vi "log analysis_gps.vi"() -> ()   [LabVIEW 2019] (continued)
2107,281532.450,02000000,471d,15824;INS_ALIGNMENT_COMPLETE,INS_RTKFIXED,37.37125529086,126.72205393210,7.8208,22.3000,-0.0380,0.2964,0.0024,-1.066354382,0.654899534,89.120116128,0.4138,0.2906,0.5321,0.1104,0.0921,0.0766,0.1807,0.1849,5.1689,0f000001,0*be946886\n\t", "INSPVAXA,USB3,0,47.5,FINESTEERING,2107,281532.950,02000000,471d,15824;INS_ALIGNMENT_COMPLETE,INS_RTKFIXED,37.37125523061,126.72205555403,7.8287,22.3000,-0.0378,0.2817,0.0049,-1.169453281,0.642583735,89.146408526,0.4138,0.2906,0.5321,0.1104,0.0921,0.0766,0.1807,0.1849,5.1689,0f000001,0*6f8607ae\n\t", "INSPVAXA,USB3,0,48.5,FINESTEERING,2107,281533.450,02000000,471d,15824;INS_ALIGNMENT_COMPLETE,INS_RTKFIXED,37.37125517665,126.72205724840,7.8341,22.3000,-0.0370,0.2921,0.0139,-1.096637131,0.532202635,89.160335545,0.4113,0.2846,0.5267,0.1101,0.0906,0.0761,0.1804,0.1849,5.1704,0f000001,0*30c8b167\n\t", "INSPVAXA,USB3,0,48.5,FINESTEERING,2107,281533.950,02000000,471d,15824;INS_ALIGNMENT_COMPLETE,INS_RTKFIXED,37.37125511841,126.72205890911,7.8393,22.3000,-0.0280,0.2944,0.0195,-1.130148525,0.576717755,89.139209909,0.4113,0.2846,0.5267,0.1101,0.0906,0.0761,0.1804,0.1849,5.1704,0f000001,0*9cf16a0c\n\t", "INSPVAXA,USB3,0,49.0,FINESTEERING,2107,281534.450,02000000,471d,15824;INS_ALIGNMENT_COMPLETE,INS_RTKFIXED,37.37125507853,126.72206052520,7.8451,22.3000,-0.0278,0.2839,0.0233,-1.120245446,0.696634414,89.152346595,0.4098,0.2808,0.5226,0.1101,0.0900,0.0757,0.1802,0.1849,5.1715,0f000001,0*4ae7b9de\n\t", "INSPVAXA,USB3,0,48.5,FINESTEERING,2107,281535.450,02000000,471d,15824;INS_ALIGNMENT_COMPLETE,INS_RTKFIXED,37.37125500223,126.72206378998,7.8595,22.3000,-0.0263,0.2848,0.0309,-1.021616386,0.668311678,89.031237589,0.4086,0.2786,0.5193,0.1098,0.0898,0.0755,0.1801,0.1849,5.1718,0f000001,0*96cd35cb\n\t", "INSPVAXA,USB3,0,48.5,FINESTEERING,2107,281535.950,02000000,471d,15824;INS_ALIGNMENT_COMPLETE,INS_RTKFIXED,37.37125496736,126.72206538562,7.8673,22.3000,-0.0208,0.2826,0.0283,-0.984984816,0.649258027,88.926389870,0.4086,0.2786,0.5193,0.1098,0.0898,0.0755,0.1801,0.1849,5.1718,0f000001,0*d651761b\n\t", "INSPVAXA,USB3,0,43.0,FINESTEERING,2107,281536.450,02000000,471d,15824;INS_ALIGNMENT_COMPLETE,INS_RTKFIXED,37.37125494902,126.72206698066,7.8731,22.3000,-0.0263,0.2809,0.0211,-1.040366850,0.673880913,88.812825832,0.4080,0.2774,0.5168,0.1098,0.0898,0.0754,0.1801,0.1849,5.1719,0f000001,0*bc17f841\n\t", "INSPVAXA,USB3,0,43.0,FINESTEERING,2107,281536.950,02000000,471d,15824;INS_ALIGNMENT_COMPLETE,INS_RTKFIXED,37.37125492336,126.72206864315,7.8782,22.3000,-0.0243,0.2721,0.0164,-1.054954219,0.518295221,88.745495992,0.4080,0.2774,0.5168,0.1098,0.0898,0.0754,0.1801,0.1849,5.1719,0f000001,0*93a4c9d5\n\t", "INSPVAXA,USB3,0,49.5,FINESTEERING,2107,281537.450,02000000,471d,15824;INS_ALIGNMENT_COMPLETE,INS_RTKFIXED,37.37125492115,126.72207026375,7.8826,22.3000,-0.0312,0.2819,0.0093,-1.140326521,0.505680826,88.594443704,0.4075,0.2769,0.5150,0.1098,0.0900,0.0754,0.1800,0.1848,5.1716,0f000001,0*0036ae1b\n\t", "INSPVAXA,USB3,0,49.5,FINESTEERING,2107,281537.950,02000000,471d,15824;INS_ALIGNMENT_COMPLETE,INS_RTKFIXED,37.37125491697,126.72207184054,7.8872,22.3000,-0.0272,0.2819,0.0040,-1.130976236,0.507935776,88.476377303,0.4075,0.2769,0.5150,0.1098,0.0900,0.0754,0.1800,0.1848,5.1716,0f000001,0*f6fa546b\n\t", "INSPVAXA,USB3,0,49.5,FINESTEERING,2107,281538.450,02000000,471d,15824;INS_ALIGNMENT_COMPLETE,INS_RTKFIXED,37.37125491162,126.72207343326,7.8918,22.3000,-0.0245,0.2815,0.0124,-1.153453506,0.493104111,88.435314047,0.4072,0.2765,0.5135,0.1099,0.0900,0.0754,0.1800,0.1848,5.1710,0f000001,0*5ae8f9c6\n\t", "INSPVAXA,USB3,0,49.5,FINESTEERING,2107,281538.950,02000000,471d,15824;INS_ALIGNMENT_COMPLETE,INS_RTKFIXED,37.37125490028,126.72207504818,7.8968,22.3000,-0.0236,0.2833,0.0059,-1.091251980,0.482969465,88.379863366,0.4072,0.2765,0.5135,0.1099,0.0900,0.0754,0.1800,0.1848,5.1710,0f000001,0*2ba689f0\n\t", "INSPVAXA,USB3,0,48.5,FINESTEERING,2107,281539.450,02000000,471d,15824;INS_ALIGNMENT_COMPLETE,INS_RTKFIXED,37.37125490824,126.72207664117,7.9004,22.3000,-0.0216,0.2784,0.0079,-1.109314476,0.482411091,88.340192961,0.4069,0.2763,0.5124,0.1098,0.0900,0.0754,0.1799,0.1848,5.1698,0f000001,0*8761aced\n\t", "INSPVAXA,USB3,0,48.5,FINESTEERING,2107,281539.950,02000000,471d,15824;INS_ALIGNMENT_COMPLETE,INS_RTKFIXED,37.37125492237,126.72207822482,7.9044,22.3000,-0.0192,0.2821,0.0128,-1.302544684,0.456729396,88.350488881,0.4069,0.2763,0.5124,0.1098,0.0900,0.0754,0.1799,0.1848,5.1698,0f000001,0*d36670cb\n\t", "INSPVAXA,USB3,0,49.0,FINESTEERING,2107,281540.450,02000000,471d,15824;INS_ALIGNMENT_COMPLETE,INS_RTKFIXED,37.37125492050,126.72207986895,7.9075,22.3000,-0.0253,0.2731,0.0097,-1.293452361,0.411042124,88.411048342,0.4069,0.2763,0.5116,0.1099,0.0902,0.0754,0.1799,0.1848,5.1684,0f000001,0*2b0ddc64\n\t", "INSPVAXA,USB3,0,48.5,FINESTEERING,2107,281541.950,02000000,471d,15824;INS_ALIGNMENT_COMPLETE,INS_RTKFIXED,37.37125486975,126.72208463852,7.9183,22.3000,-0.0254,0.2525,0.0080,-1.001794555,0.208047593,88.595435121,0.4068,0.2761,0.5109,0.1098,0.0900,0.0754,0.1799,0.1848,5.1663,0f000001,0*dcb79567\n\t", "INSPVAXA,USB3,0,49.0,FINESTEERING,2107,281542.450,02000000,471d,15824;INS_ALIGNMENT_COMPLETE,INS_RTKFIXED,37.37125484773,126.72208610696,7.9206,22.3000,-0.0083,0.3427,0.0268,-0.912942470,0.207155867,88.931332893,0.4067,0.2761,0.5105,0.1096,0.0899,0.0754,0.1798,0.1848,5.1642,0f000001,0*e5dcf027\n\t", "INSPVAXA,USB3,0,49.5,FINESTEERING,2107,281543.950,02000000,471d,15824;INS_ALIGNMENT_COMPLETE,INS_RTKFIXED,37.37125492276,126.72209111825,7.9296,22.3000,0.0316,0.2804,0.0153,-0.692370784,0.020659336,82.875038153,0.4068,0.2761,0.5102,0.1095,0.0899,0.0754,0.1798,0.1847,5.1628,0f000001,0*67f5d293\n\t", "INSPVAXA,USB3,0,50.0,FINESTEERING,2107,281544.450,02000000,471d,15824;INS_ALIGNMENT_COMPLETE,INS_RTKFIXED,37.37125505566,126.72209271509,7.9316,22.3000,0.0505,0.2738,0.0268,-0.616767786,0.154143258,78.067707223,0.4067,0.2763,0.5098,0.1099,0.0900,0.0754,0.1797,0.1847,5.1619,0f000001,0*4337cbac\n\t", "INSPVAXA,USB3,0,47.5,FINESTEERING,2107,281545.450,02000000,471d,15824;INS_ALIGNMENT_COMPLETE,INS_RTKFIXED,37.37125567911,126.72209586319,7.9361,22.3000,0.0734,0.2704,0.0174,-0.731540413,0.133149102,70.486374677,0.4064,0.2767,0.5097,0.1103,0.0911,0.0753,0.1798,0.1847,5.1599,0f000001,0*4759ac49\n\t", "INSPVAXA,USB3,0,47.5,FINESTEERING,2107,281545.950,02000000,471d,15824;INS_ALIGNMENT_COMPLETE,INS_RTKFIXED,37.37125607129,126.72209738757,7.9408,22.3000,0.0944,0.2605,0.0183,-0.696019275,0.088406772,68.352521751,0.4064,0.2767,0.5097,0.1103,0.0911,0.0753,0.1798,0.1847,5.1599,0f000001,0*d303d9f5\n\t", "INSPVAXA,USB3,0,49.0,FINESTEERING,2107,281546.450,02000000,471d,15824;INS_ALIGNMENT_COMPLETE,INS_RTKFIXED,37.37125652974,126.72209892700,7.9445,22.3000,0.1147,0.2632,0.0224,-0.803440869,0.020202834,66.760557028,0.4064,0.2770,0.5100,0.1115,0.0928,0.0753,0.1798,0.1846,5.1557,0f000001,0*6d000163\n\t", "INSPVAXA,USB3,0,51.5,FINESTEERING,2107,281547.950,02000000,471d,15824;INS_ALIGNMENT_COMPLETE,INS_RTKFIXED,37.37125797695,126.72210352475,7.9421,22.3000,0.1103,0.2645,0.0073,-1.143829533,0.094704547,65.656045982,0.4068,0.2775,0.5101,0.1136,0.0952,0.0753,0.1797,0.1843,5.1506,0f000001,0*3e76ed6a\n\t", "INSPVAXA,USB3,0,46.5,FINESTEERING,2107,281548.450,02000000,471d,15824;INS_ALIGNMENT_COMPLETE,INS_RTKFIXED,37.37125842194,126.72210499734,7.9414,22.3000,0.0987,0.2565,0.0113,-1.211419516,0.114110023,65.814844612,0.4000,0.2752,0.5002,0.1145,0.0964,0.0745,0.1794,0.1832,5.1447,0f000001,0*e7619ae9\n\t", "INSPVAXA,USB3,0,50.0,FINESTEERING,2107,281550.450,02000000,471d,15824;INS_ALIGNMENT_COMPLETE,INS_RTKFIXED,37.37126014909,126.72211137085,7.9382,22.3000,0.0775,0.2990,0.0098,-1.324688179,-0.327901204,70.475818892,0.4093,0.2808,0.5055,0.1189,0.0988,0.0751,0.1779,0.1804,5.1364,0f000001,0*808235da\n\t", "INSPVAXA,USB3,0,50.0,FINESTEERING,2107,281550.950,02000000,471d,15824;INS_ALIGNMENT_COMPLETE,INS_RTKFIXED,37.37126045851,126.72211301062,7.9366,22.3000,0.0692,0.2949,0.0149,-1.528450256,-0.256130387,73.623851068,0.4093,0.2808,0.5055,0.1189,0.0988,0.0751,0.1779,0.1804,5.1364,0f000001,0*9b441f42\n\t", "INSPVAXA,USB3,0,50.5,FINESTEERING,2107,281551.450,02000000,471d,15824;INS_ALIGNMENT_COMPLETE,INS_RTKFIXED,37.37126071585,126.72211464730,7.9349,22.3000,0.0461,0.2986,0.0130,-1.521992533,-0.266379838,76.609836903,0.4123,0.2823,0.5064,0.1185,0.0974,0.0752,0.1766,0.1780,5.1359,0f000001,0*10c7b170\n\t", "INSPVAXA,USB3,0,46.0,FINESTEERING,2107,281553.450,02000000,471d,15824;INS_ALIGNMENT_COMPLETE,INS_RTKFIXED,37.37126103128,126.72212124839,7.9298,22.3000,-0.0140,0.3127,0.0103,-1.123324065,0.508186608,86.475443339,0.4150,0.2827,0.5081,0.1139,0.0931,0.0752,0.1739,0.1735,5.1368,0f000001,0*51a33212\n\t", "INSPVAXA,USB3,0,46.0,FINESTEERING,2107,281553.950,02000000,471d,15824;INS_ALIGNMENT_COMPLETE,INS_RTKFIXED,37.37126097435,126.72212290595,7.9280,22.3000,-0.0108,0.3087,0.0193,-0.994058231,0.235221833,88.104277640,0.4150,0.2827,0.5081,0.1139,0.0931,0.0752,0.1739,0.1735,5.1368,0f000001,0*a2074ee6\n\t", "INSPVAXA,USB3,0,47.5,FINESTEERING,2107,281557.450,02000000,471d,15824;INS_ALIGNMENT_COMPLETE,INS_RTKFIXED,37.37126007127,126.72213399175,7.9228,22.3000,-0.0436,0.2932,0.0085,-0.364989974,-0.412142636,90.870623018,0.4100,0.2787,0.5090,0.1093,0.0914,0.0751,0.1708,0.1703,5.1179,0f000001,0*5c4f0bd9\n\t", "INSPVAXA,USB3,0,46.0,FINESTEERING,2107,281558.450,02000000,471d,15824;INS_ALIGNMENT_COMPLETE,INS_RTKFIXED,37.37125980811,126.72213741354,7.9201,22.3000,-0.0396,0.2827,0.0144,-0.665732137,-0.749833579,90.834139291,0.4087,0.2784,0.5089,0.1102,0.0917,0.0750,0.1706,0.1703,5.1108,0f000001,0*c48606ec\n\t", "INSPVAXA,USB3,0,46.0,FINESTEERING,2107,281558.950,02000000,471d,15824;INS_ALIGNMENT_COMPLETE,INS_RTKFIXED,37.37125968631,126.72213896635,7.9182,22.3000,-0.0389,0.2938,0.0155,-0.920394419,-0.718289974,90.450245046,0.4087,0.2784,0.5089,0.1102,0.0917,0.0750,0.1706,0.1703,5.1108,0f000001,0*246e9289\n\t", "INSPVAXA,USB3,0,48.5,FINESTEERING,2107,281582.000,02000000,471d,15824;INS_ALIGNMENT_COMPLETE,INS_RTKFIXED,37.37125926697,126.72221314243,7.9638,22.3000,0.0065,0.2832,0.0220,-0.844956483,-0.026158862,84.896486231,0.4081,0.2757,0.5033,0.1092,0.0895,0.0749,0.1683,0.1693,5.0877,0f000001,0*999c2cb4\n\t", "INSPVAXA,USB3,0,45.5,FINESTEERING,2107,281585.000,02000000,471d,15824;INS_ALIGNMENT_COMPLETE,INS_RTKFIXED,37.37125940272,126.72222284495,7.9649,22.3000,-0.0095,0.2865,0.0182,-0.747268326,0.234159981,85.317572401,0.4076,0.2752,0.5032,0.1094,0.0898,0.0748,0.1683,0.1693,5.0921,0f000001,0*05cc0da4\n\t", "INSPVAXA,USB3,0,49.5,FINESTEERING,2107,281585.500,02000000,471d,15824;INS_ALIGNMENT_COMPLETE,INS_RTKFIXED,37.37125941547,126.72222448778,7.9662,22.3000,-0.0142,0.2884,0.0124,-0.699076432,0.369703687,85.497806859,0.4078,0.2753,0.5032,0.1096,0.0899,0.0748,0.1684,0.1693,5.0937,0f000001,0*7e52f1b7\n\t", "INSPVAXA,USB3,0,49.5,FINESTEERING,2107,281586.500,02000000,471d,15824;INS_ALIGNMENT_COMPLETE,INS_RTKFIXED,37.37125940571,126.72222789541,7.9680,22.3000,0.0030,0.3079,0.0233,-0.562980027,0.263238278,85.915106652,0.4081,0.2752,0.5032,0.1097,0.0899,0.0748,0.1684,0.1692,5.0953,0f000001,0*7d04a5bf\n\t", "INSPVAXA,USB3,0,49.5,FINESTEERING,2107,281587.000,02000000,471d,15824;INS_ALIGNMENT_COMPLETE,INS_RTKFIXED,37.37125938358,126.72222955995,7.9677,22.3000,-0.0088,0.3126,0.0171,-0.528697229,0.195556365,86.199096589,0.4081,0.2752,0.5032,0.1097,0.0899,0.0748,0.1684,0.1692,5.0953,0f000001,0*98856aba\n\t", "INSPVAXA,USB3,0,47.0,FINESTEERING,2107,281587.500,02000000,471d,15824;INS_ALIGNMENT_COMPLETE,INS_RTKFIXED,37.37125935739,126.72223128487,7.9668,22.3000,-0.0030,0.3090,0.0190,-0.470354496,0.052583887,86.493869068,0.4079,0.2752,0.5030,0.1098,0.0899,0.0747,0.1684,0.1690,5.0969,0f000001,0*c1a2a853\n\t", "INSPVAXA,USB3,0,45.5,FINESTEERING,2107,281590.500,02000000,471d,15824;INS_ALIGNMENT_COMPLETE,INS_RTKFIXED,37.37125890881,126.72224121064,7.9541,22.3000,-0.0384,0.3088,0.0049,0.158198742,0.001802096,88.889148367,0.4071,0.2753,0.5028,0.1097,0.0897,0.0747,0.1683,0.1686,5.0995,0f000001,0*955ddbd0\n\t", "INSPVAXA,USB3,0,45.5,FINESTEERING,2107,281591.000,02000000,471d,15824;INS_ALIGNMENT_COMPLETE,INS_RTKFIXED,37.37125878805,126.72224284394,7.9517,22.3000,-0.0402,0.3180,0.0042,0.353980649,0.071732685,89.195409994,0.4071,0.2753,0.5028,0.1097,0.0897,0.0747,0.1683,0.1686,5.0995,0f000001,0*1c59d57f\n\t", "INSPVAXA,USB3,0,48.0,FINESTEERING,2107,281591.500,02000000,471d,15824;INS_ALIGNMENT_COMPLETE,INS_RTKFIXED,37.37125869638,126.72224442366,7.9492,22.3000,-0.0439,0.3158,0.0021,0.440194436,0.083978033,89.508465675,0.4069,0.2753,0.5025,0.1096,0.0897,0.0747,0.1683,0.1685,5.0994,0f000001,0*cd52a6fa\n\t", "INSPVAXA,USB3,0,49.0,FINESTEERING,2107,281592.500,02000000,471d,15824;INS_ALIGNMENT_COMPLETE,INS_RTKFIXED,37.37125852305,126.72224758487,7.9467,22.3000,-0.0419,0.2989,0.0081,0.241164768,-0.091182939,89.866254951,0.4067,0.2753,0.5023,0.1093,0.0896,0.0746,0.1683,0.1684,5.0986,0f000001,0*7410d7bd\n\t", "INSPVAXA,USB3,0,49.0,FINESTEERING,2107,281593.000,02000000,471d,15824;INS_ALIGNMENT_COMPLETE,INS_RTKFIXED,37.37125843294,126.72224909789,7.9463,22.3000,-0.0494,0.2967,0.0111,0.084019586,0.037300325,90.030415864,0.4067,0.2753,0.5023,0.1093,0.0896,0.0746,0.1683,0.1684,5.0986,0f000001,0*0c6e6e15\n\t", "INSPVAXA,USB3,0,47.0,FINESTEERING,2107,281593.500,02000000,471d,15824;INS_ALIGNMENT_COMPLETE,INS_RTKFIXED,37.37125834817,126.72225064621,7.9448,22.3000,-0.0530,0.2881,0.0083,-0.027403360,0.078247142,90.176817811,0.4066,0.2752,0.5020,0.1093,0.0894,0.0746,0.1682,0.1684,5.0980,0f000001,0*f779539b\n\t", "INSPVAXA,USB3,0,49.0,FINESTEERING,2107,281594.500,02000000,471d,15824;INS_ALIGNMENT_COMPLETE,INS_RTKFIXED,37.37125815716,126.72225388561,7.9395,22.3000,-0.0550,0.3023,0.0057,-0.022782572,-0.170277850,90.320435048,0.4065,0.2750,0.5018,0.1093,0.0894,0.0746,0.1682,0.1684,5.0981,0f000001,0*f8af8c2b\n\t", "INSPVAXA,USB3,0,49.0,FINESTEERING,2107,281595.000,02000000,471d,15824;INS_ALIGNMENT_COMPLETE,INS_RTKFIXED,37.37125806903,126.72225552746,7.9370,22.3000,-0.0572,0.3021,0.0033,-0.060546798,-0.376099237,90.424899163,0.4065,0.2750,0.5018,0.1093,0.0894,0.0746,0.1682,0.1684,5.0981,0f000001,0*15f57f01\n\t", "INSPVAXA,USB3,0,49.0,FINESTEERING,2107,281596.000,02000000,471d,15824;INS_ALIGNMENT_COMPLETE,INS_RTKFIXED,37.37125790124,126.72225886435,7.9333,22.3000,-0.0466,0.2890,0.0127,-0.410308498,-0.648762908,90.450935074,0.4065,0.2747,0.5016,0.1095,0.0895,0.0746,0.1681,0.1684,5.0986,0f000001,0*6915a645\n\t", "INSPVAXA,USB3,0,49.5,FINESTEERING,2107,281596.500,02000000,471d,15824;INS_ALIGNMENT_COMPLETE,INS_RTKFIXED,37.37125781382,126.72226046483,7.9311,22.3000,-0.0418,0.2833,0.0090,-0.435085374,-0.543120061,90.230742577,0.4063,0.2745,0.5015,0.1095,0.0898,0.0746,0.1681,0.1684,5.0990,0f000001,0*49551541\n\t", "INSPVAXA,USB3,0,49.5,FINESTEERING,2107,281597.000,02000000,471d,15824;INS_ALIGNMENT_COMPLETE,INS_RTKFIXED,37.37125771210,126.72226205669,7.9296,22.3000,-0.0419,0.3034,0.0146,-0.176475968,-0.465211146,89.900752535,0.4063,0.2745,0.5015,0.1095,0.0898,0.0746,0.1681,0.1684,5.0990,0f000001,0*aa558b24\n\t", "INSPVAXA,USB3,0,50.0,FINESTEERING,2107,281597.500,02000000,471d,15824;INS_ALIGNMENT_COMPLETE,INS_RTKFIXED,37.37125762620,126.72226364430,7.9270,22.3000,-0.0431,0.2944,0.0123,-0.034850827,-0.383453655,89.494102450,0.4062,0.2742,0.5014,0.1094,0.0896,0.0746,0.1680,0.1684,5.0989,0f000001,0*eb33c8cb\n\t", "INSPVAXA,USB3,0,50.0,FINESTEERING,2107,281598.000,02000000,471d,15824;INS_ALIGNMENT_COMPLETE,INS_RTKFIXED,37.37125755430,126.72226525077,7.9232,22.3000,-0.0288,0.2974,0.0131,0.018056318,-0.346106265,89.006732847,0.4062,0.2742,0.5014,0.1094,0.0896,0.0746,0.1680,0.1684,5.0989,0f000001,0*7f8cff1a\n\t", "INSPVAXA,USB3,0,47.5,FINESTEERING,2107,281598.500,02000000,471d,15824;INS_ALIGNMENT_COMPLETE,INS_RTKFIXED,37.37125752692,126.72226686003,7.9200,22.3000,-0.0297,0.2922,-0.0044,-0.122753848,-0.350679185,88.582247328,0.4061,0.2743,0.5013,0.1093,0.0895,0.0746,0.1680,0.1684,5.0986,0f000001,0*76a956e7\n\t", "INSPVAXA,USB3,0,47.5,FINESTEERING,2107,281599.000,02000000,471d,15824;INS_ALIGNMENT_COMPLETE,INS_RTKFIXED,37.37125750157,126.72226846220,7.9172,22.3000,-0.0394,0.2975,0.0004,-0.262738431,-0.259927736,88.093141362,0.4061,0.2743,0.5013,0.1093,0.0895,0.0746,0.1680,0.1684,5.0986,0f000001,0*5a405d12\n\t", "INSPVAXA,USB3,0,47.5,FINESTEERING,2107,281599.500,02000000,471d,15824;INS_ALIGNMENT_COMPLETE,INS_RTKFIXED,37.37125749812,126.72227005344,7.9138,22.3000,-0.0467,0.2803,-0.0089,-0.269229202,-0.225074216,87.528625301,0.4063,0.2743,0.5013,0.1092,0.0896,0.0746,0.1679,0.1685,5.0987,0f000001,0*0f923b8c\n\t", "INSPVAXA,USB3,0,47.5,FINESTEERING,2107,281600.000,02000000,471d,15824;INS_ALIGNMENT_COMPLETE,INS_RTKFIXED,37.37125749625,126.72227167040,7.9096,22.3000,-0.0440,0.2738,-0.0170,-0.124807872,-0.330803531,87.082207442,0.4063,0.2743,0.5013,0.1092,0.0896,0.0746,0.1679,0.1685,5.0987,0f000001,0*844dad1a\n\t", "DUALANTENNAHEADINGA,USB3,0,49.5,FINESTEERING,2107,281600.500,02000000,d426,15824;SOL_COMPUTED,NARROW_FLOAT,-1.000000000,72.063247681,-40.725646973,0.0,273.105743408,180.000000000,\"631T\",22,8,8,8,04,00,20,23*8da2d13b\n\t", "INSPVAXA,USB3,0,49.5,FINESTEERING,2107,281601.000,02000000,471d,15824;INS_ALIGNMENT_COMPLETE,INS_RTKFIXED,37.37125751795,126.72227489272,7.9035,22.3000,-0.0358,0.2988,-0.0067,-0.198567071,-0.277392805,86.699743211,0.4065,0.2744,0.5014,0.1092,0.0895,0.0746,0.1679,0.1685,5.0988,0f000001,0*2cadf3ab\n\t", "INSPVAXA,USB3,0,48.0,FINESTEERING,2107,281601.500,02000000,471d,15824;INS_ALIGNMENT_COMPLETE,INS_RTKFIXED,37.37125754133,126.72227651684,7.9018,22.3000,-0.0303,0.2880,-0.0022,-0.260652081,-0.486725638,86.696539818,0.4068,0.2744,0.5014,0.1092,0.0895,0.0746,0.1679,0.1685,5.0994,0f000001,0*3e737448\n\t", "INSPVAXA,USB3,0,48.0,FINESTEERING,2107,281602.000,02000000,471d,15824;INS_ALIGNMENT_COMPLETE,INS_RTKFIXED,37.37125756266,126.72227812513,7.9001,22.3000,-0.0263,0.2865,-0.0045,-0.342075300,-0.515152561,86.801185345,0.4068,0.2744,0.5014,0.1092,0.0895,0.0746,0.1679,0.1685,5.0994,0f000001,0*64049b1c\n\t", "INSPVAXA,USB3,0,49.0,FINESTEERING,2107,281602.500,02000000,471d,15824;INS_ALIGNMENT_COMPLETE,INS_RTKFIXED,37.37125758385,126.72227971181,7.8988,22.3000,-0.0248,0.2942,-0.0059,-0.465449953,-0.482180985,86.903233906,0.4069,0.2744,0.5013,0.1092,0.0896,0.0746,0.1678,0.1685,5.1000,0f000001,0*df1bf2df\n\t", "INSPVAXA,USB3,0,49.0,FINESTEERING,2107,281603.000,02000000,471d,15824;INS_ALIGNMENT_COMPLETE,INS_RTKFIXED,37.37125760896,126.72228133197,7.8974,22.3000,-0.0248,0.2888,-0.0003,-0.623364268,-0.535478966,87.043420803,0.4069,0.2744,0.5013,0.1092,0.0896,0.0746,0.1678,0.1685,5.1000,0f000001,0*b0d9f6c7\n\t", "INSPVAXA,USB3,0,49.5,FINESTEERING,2107,281603.500,02000000,471d,15824;INS_ALIGNMENT_COMPLETE,INS_RTKFIXED,37.37125762014,126.72228294521,7.8952,22.3000,-0.0259,0.2842,0.0002,-0.657593864,-0.460325437,87.196665885,0.4072,0.2744,0.5014,0.1092,0.0897,0.0746,0.1678,0.1686,5.1007,0f000001,0*32d6fd63\n\t", "INSPVAXA,USB3,0,49.5,FINESTEERING,2107,281604.000,02000000,471d,15824;INS_ALIGNMENT_COMPLETE,INS_RTKFIXED,37.37125761729,126.72228447790,7.8935,22.3000,-0.0300,0.2898,-0.0081,-0.656830012,-0.299740331,87.333790648,0.4072,0.2744,0.5014,0.1092,0.0897,0.0746,0.1678,0.1686,5.1007,0f000001,0*76a7715c\n\t", "INSPVAXA,USB3,0,44.5,FINESTEERING,2107,281604.500,02000000,471d,15824;INS_ALIGNMENT_COMPLETE,INS_RTKFIXED,37.37125762223,126.72228607343,7.8940,22.3000,-0.0219,0.2910,-0.0031,-0.589546235,-0.368304883,87.506526746,0.4072,0.2745,0.5015,0.1092,0.0897,0.0746,0.1678,0.1685,5.1010,0f000001,0*388a7a2d\n\t", "INSPVAXA,USB3,0,44.5,FINESTEERING,2107,281605.000,02000000,471d,15824;INS_ALIGNMENT_COMPLETE,INS_RTKFIXED,37.37125762402,126.72228771590,7.8945,22.3000,-0.0210,0.3023,-0.0017,-0.565411059,-0.344280902,87.705183727,0.4072,0.2745,0.5015,0.1092,0.0897,0.0746,0.1678,0.1685,5.1010,0f000001,0*43df75d8\n\t", "INSPVAXA,USB3,0,49.5,FINESTEERING,2107,281605.500,02000000,471d,15824;INS_ALIGNMENT_COMPLETE,INS_RTKFIXED,37.37125763713,126.72228942548,7.8937,22.3000,-0.0187,0.2984,0.0018,-0.682644637,-0.329022185,87.922528604,0.4076,0.2746,0.5016,0.1093,0.0897,0.0746,0.1678,0.1685,5.1013,0f000001,0*79d36c9f\n\t", "INSPVAXA,USB3,0,49.5,FINESTEERING,2107,281606.000,02000000,471d,15824;INS_ALIGNMENT_COMPLETE,INS_RTKFIXED,37.37125764382,126.72229106534,7.8933,22.3000,-0.0223,0.2951,0.0001,-0.712476765,-0.315068530,88.171988719,0.4076,0.2746,0.5016,0.1093,0.0897,0.0746,0.1678,0.1685,5.1013,0f000001,0*a3ebc004\n\t", "INSPVAXA,USB3,0,50.0,FINESTEERING,2107,281606.500,02000000,471d,15824;INS_ALIGNMENT_COMPLETE,INS_RTKFIXED,37.37125763803,126.72229270568,7.8917,22.3000,-0.0150,0.3037,-0.0036,-0.690294492,-0.219977588,88.452886392,0.4077,0.2746,0.5015,0.1093,0.0897,0.0746,0.1678,0.1685,5.1018,0f000001,0*e1d1f507\n\t", "INSPVAXA,USB3,0,50.0,FINESTEERING,2107,281607.000,02000000,471d,15824;INS_ALIGNMENT_COMPLETE,INS_RTKFIXED,37.37125762815,126.72229434491,7.8899,22.3000,-0.0081,0.2973,0.0070,-0.653085669,-0.059361264,88.754704590,0.4077,0.2746,0.5015,0.1093,0.0897,0.0746,0.1678,0.1685,5.1018,0f000001,0*aec8b341\n\t", "INSPVAXA,USB3,0,50.5,FINESTEERING,2107,281607.500,02000000,471d,15824;INS_ALIGNMENT_COMPLETE,INS_RTKFIXED,37.37125761017,126.72229595804,7.8881,22.3000,-0.0137,0.2967,-0.0028,-0.749913481,-0.074231806,89.214794289,0.4080,0.2746,0.5014,0.1093,0.0897,0.0746,0.1678,0.1684,5.1022,0f000001,0*37633f72\n\t", "DUALANTENNAHEADINGA,USB3,0,50.5,FINESTEERING,2107,281608.000,02000000,d426,15824;SOL_COMPUTED,NARROW_FLOAT,-1.000000000,78.494079590,-41.424682617,0.0,180.103469849,180.000000000,\"631T\",21,10,10,8,04,00,20,23*2f530816\n\t", "INSPVAXA,USB3,0,45.0,FINESTEERING,2107,281608.500,02000000,471d,15824;INS_ALIGNMENT_COMPLETE,INS_RTKFIXED,37.37125753147,126.72229922656,7.8853,22.3000,-0.0283,0.3023,-0.0044,-0.783072091,-0.564713007,90.330728689,0.4085,0.2746,0.5015,0.1092,0.0897,0.0746,0.1678,0.1684,5.1027,0f000001,0*a72eaeae\n\t", "INSPVAXA,USB3,0,45.0,FINESTEERING,2107,281609.000,02000000,471d,15824;INS_ALIGNMENT_COMPLETE,INS_RTKFIXED,37.37125746019,126.72230086669,7.8844,22.3000,-0.0388,0.2946,-0.0124,-0.730333376,-0.851088036,90.998664332,0.4085,0.2746,0.5015,0.1092,0.0897,0.0746,0.1678,0.1684,5.1027,0f000001,0*4f9cf076\n\t", "INSPVAXA,USB3,0,49.5,FINESTEERING,2107,281609.500,02000000,471d,15824;INS_ALIGNMENT_COMPLETE,INS_RTKFIXED,37.37125736767,126.72230251871,7.8837,22.3000,-0.0246,0.2829,-0.0110,-0.778570113,-1.137011227,91.636107067,0.4086,0.2746,0.5016,0.1092,0.0896,0.0746,0.1678,0.1683,5.1032,0f000001,0*f38f9db8\n\t", "INSPVAXA,USB3,0,49.5,FINESTEERING,2107,281610.000,02000000,471d,15824;INS_ALIGNMENT_COMPLETE,INS_RTKFIXED,37.37125727212,126.72230414457,7.8824,22.3000,-0.0153,0.2788,0.0009,-0.850299061,-1.150279108,92.167621233,0.4086,0.2746,0.5016,0.1092,0.0896,0.0746,0.1678,0.1683,5.1032,0f000001,0*9822d498\n\t", "DUALANTENNAHEADINGA,USB3,0,49.5,FINESTEERING,2107,281610.500,02000000,d426,15824;SOL_COMPUTED,L1_FLOAT,-1.000000000,84.036529541,-51.585266113,0.0,298.644531250,180.000000000,\"631T\",20,8,8,8,04,00,20,23*45ddee6b\n\t", "DUALANTENNAHEADINGA,USB3,0,49.5,FINESTEERING,2107,281611.000,02000000,d426,15824;SOL_COMPUTED,L1_FLOAT,-1.000000000,84.902954102,-51.688964844,0.0,297.235992432,180.000000000,\"631T\",20,8,8,8,04,00,20,23*432775c3\n\t", "DUALANTENNAHEADINGA,USB3,0,48.0,FINESTEERING,2107,281611.500,02000000,d426,15824;SOL_COMPUTED,NARROW_FLOAT,-1.000000000,80.569839478,-43.681274414,0.0,202.652938843,180.000000000,\"631T\",19,9,9,7,04,00,20,23*350caf71\n\t", "INSPVAXA,USB3,0,48.0,FINESTEERING,2107,281612.000,02000000,471d,15824;INS_ALIGNMENT_COMPLETE,INS_RTKFIXED,37.37125679959,126.72231051276,7.8723,22.3000,-0.0152,0.2724,0.0005,-0.625404023,-0.811400183,93.401020148,0.4082,0.2744,0.5017,0.1093,0.0896,0.0746,0.1677,0.1683,5.1044,0f000001,0*fa2c836e\n\t", "INSPVAXA,USB3,0,46.0,FINESTEERING,2107,281612.500,02000000,471d,15824;INS_ALIGNMENT_COMPLETE,INS_RTKFIXED,37.37125664766,126.72231208737,7.8703,22.3000,-0.0138,0.2840,-0.0007,-0.548027474,-0.764885305,93.580702157,0.4082,0.2744,0.5017,0.1093,0.0896,0.0746,0.1677,0.1683,5.1050,0f000001,0*f22f9aa7\n\t", "INSPVAXA,USB3,0,46.0,FINESTEERING,2107,281613.000,02000000,471d,15824;INS_ALIGNMENT_COMPLETE,INS_RTKFIXED,37.37125650617,126.72231359099,7.8684,22.3000,-0.0180,0.2849,-0.0146,-0.566383475,-0.626492168,93.731901396,0.4082,0.2744,0.5017,0.1093,0.0896,0.0746,0.1677,0.1683,5.1050,0f000001,0*d3b26d7f\n\t", "DUALANTENNAHEADINGA,USB3,0,45.0,FINESTEERING,2107,281613.500,02000000,d426,15824;SOL_COMPUTED,L1_FLOAT,-1.000000000,83.088043213,-56.739044189,0.0,275.930023193,180.000000000,\"631T\",19,6,6,6,04,00,20,03*7fa5a20d\n\t", "DUALANTENNAHEADINGA,USB3,0,45.0,FINESTEERING,2107,281614.000,02000000,d426,15824;SOL_COMPUTED,L1_FLOAT,-1.000000000,82.710388184,-57.006988525,0.0,271.422698975,180.000000000,\"631T\",19,6,6,6,04,00,20,03*129b017c\n\t", "DUALANTENNAHEADINGA,USB3,0,46.5,FINESTEERING,2107,281614.500,02000000,d426,15824;SOL_COMPUTED,L1_FLOAT,-1.000000000,82.445899963,-51.127838135,0.0,347.003540039,180.000000000,\"631T\",19,6,6,6,04,00,20,03*63fc53d7\n\t", "DUALANTENNAHEADINGA,USB3,0,46.5,FINESTEERING,2107,281615.000,02000000,d426,15824;SOL_COMPUTED,L1_FLOAT,-1.000000000,81.371170044,-46.344207764,0.0,346.866485596,180.000000000,\"631T\",19,6,6,6,04,00,20,03*e0ade60f\n\t", "DUALANTENNAHEADINGA,USB3,0,50.5,FINESTEERING,2107,281615.500,02000000,d426,15824;SOL_COMPUTED,NARROW_FLOAT,-1.000000000,80.817100525,-47.001037598,0.0,207.681015015,180.000000000,\"631T\",20,6,6,6,04,00,20,03*9d84b137\n\t", "DUALANTENNAHEADINGA,USB3,0,50.5,FINESTEERING,2107,281616.000,02000000,d426,15824;SOL_COMPUTED,NARROW_FLOAT,-1.000000000,81.509902954,-49.725524902,0.0,216.669723511,180.000000000,\"631T\",20,6,6,6,04,00,20,03*6356a6a7\n\t", "INSPVAXA,USB3,0,47.5,FINESTEERING,2107,281616.500,02000000,471d,15824;INS_ALIGNMENT_COMPLETE,INS_RTKFIXED,37.37125540027,126.72232487564,7.8689,22.3000,-0.0235,0.2865,-0.0155,-0.776428369,-0.126871761,92.710705612,0.4096,0.2747,0.5015,0.1097,0.0898,0.0746,0.1674,0.1681,5.1098,0f000001,0*a35ee19b\n\t", "DUALANTENNAHEADINGA,USB3,0,47.5,FINESTEERING,2107,281617.000,02000000,d426,15824;SOL_COMPUTED,NARROW_FLOAT,-1.000000000,83.135253906,-45.598937988,0.0,198.452239990,180.000000000,\"631T\",19,7,7,6,04,00,20,03*722e59f8\n\t", "INSPVAXA,USB3,0,49.0,FINESTEERING,2107,281617.500,02000000,471d,15824;INS_ALIGNMENT_COMPLETE,INS_RTKFIXED,37.37125515068,126.72232806022,7.8714,22.3000,-0.0152,0.2731,0.0045,-0.723483690,-0.404647650,90.811415851,0.4097,0.2748,0.5015,0.1095,0.0898,0.0746,0.1673,0.1681,5.1105,0f000001,0*086db8d4\n\t", "INSPVAXA,USB3,0,49.0,FINESTEERING,2107,281618.000,02000000,471d,15824;INS_ALIGNMENT_COMPLETE,INS_RTKFIXED,37.37125505743,126.72232965261,7.8715,22.3000,-0.0112,0.2768,-0.0033,-0.719605917,-0.592487460,89.836730545,0.4097,0.2748,0.5015,0.1095,0.0898,0.0746,0.1673,0.1681,5.1105,0f000001,0*7f7a4829\n\t", "DUALANTENNAHEADINGA,USB3,0,49.5,FINESTEERING,2107,281618.500,02000000,d426,15824;SOL_COMPUTED,L1_FLOAT,-1.000000000,81.985870361,-51.294281006,0.0,269.498687744,180.000000000,\"631T\",17,8,8,8,04,00,20,23*d2afce59\n\t", "DUALANTENNAHEADINGA,USB3,0,49.5,FINESTEERING,2107,281619.000,02000000,d426,15824;SOL_COMPUTED,L1_FLOAT,-1.000000000,81.329711914,-49.084411621,0.0,261.078948975,180.000000000,\"631T\",18,8,8,8,04,00,20,23*0738c36d\n\t", "DUALANTENNAHEADINGA,USB3,0,48.0,FINESTEERING,2107,281619.500,02000000,d426,15824;SOL_COMPUTED,NARROW_FLOAT,-1.000000000,83.428977966,-43.865173340,0.0,179.560241699,180.000000000,\"631T\",20,9,9,8,04,00,20,23*fb7ce078\n\t", "DUALANTENNAHEADINGA,USB3,0,48.0,FINESTEERING,2107,281620.000,02000000,d426,15824;SOL_COMPUTED,NARROW_FLOAT,-1.000000000,83.177322388,-43.462402344,0.0,179.866409302,180.000000000,\"631T\",19,9,9,8,04,00,20,23*b83e1f1b\n\t", "DUALANTENNAHEADINGA,USB3,0,44.5,FINESTEERING,2107,281620.500,02000000,d426,15824;SOL_COMPUTED,NARROW_FLOAT,-1.000000000,82.434860229,-53.334503174,0.0,202.841445923,166.629974365,\"631T\",18,8,8,8,04,00,20,23*e81d707d\n\t", "INSPVAXA,USB3,0,44.5,FINESTEERING,2107,281621.000,02000000,471d,15824;INS_ALIGNMENT_COMPLETE,INS_RTKFIXED,37.37125484776,126.72233928465,7.8682,22.3000,-0.0140,0.2874,-0.0021,-0.631288099,-0.470123008,86.597817260,0.4108,0.2750,0.5022,0.1095,0.0896,0.0746,0.1671,0.1681,5.1116,0f000001,0*0301d2b2\n\t", "DUALANTENNAHEADINGA,USB3,0,47.5,FINESTEERING,2107,281621.500,02000000,d426,15824;SOL_COMPUTED,L1_FLOAT,-1.000000000,79.118186951,-47.831787109,0.0,285.028137207,180.000000000,\"631T\",21,8,8,8,04,00,20,23*eceb4aca\n\t", "DUALANTENNAHEADINGA,USB3,0,47.5,FINESTEERING,2107,281622.000,02000000,d426,15824;SOL_COMPUTED,L1_FLOAT,-1.000000000,79.215469360,-46.676361084,0.0,278.801727295,180.000000000,\"631T\",21,8,8,8,04,00,20,23*2f0de768\n\t", "DUALANTENNAHEADINGA,USB3,0,50.0,FINESTEERING,2107,281622.500,02008000,d426,15824;SOL_COMPUTED,NARROW_FLOAT,-1.000000000,81.357048035,-52.184570313,0.0,156.938522339,171.573028564,\"631T\",22,8,8,8,04,00,20,23*a9a2e0bd\n\t", "DUALANTENNAHEADINGA,USB3,0,50.0,FINESTEERING,2107,281623.000,02008000,d426,15824;SOL_COMPUTED,NARROW_FLOAT,-1.000000000,80.926651001,-50.941162109,0.0,157.099182129,180.000000000,\"631T\",22,8,8,8,04,00,20,23*29ef00a4\n\t", "DUALANTENNAHEADINGA,USB3,0,47.0,FINESTEERING,2107,281623.500,02008000,d426,15824;SOL_COMPUTED,NARROW_FLOAT,-1.000000000,74.372909546,-36.647766113,0.0,211.228378296,180.000000000,\"631T\",21,9,9,8,04,00,20,23*0d510ff3\n\t", "DUALANTENNAHEADINGA,USB3,0,47.0,FINESTEERING,2107,281624.000,02008000,d426,15824;SOL_COMPUTED,NARROW_FLOAT,-1.000000000,74.676368713,-33.559204102,0.0,205.690567017,180.000000000,\"631T\",20,9,9,8,04,00,20,23*f648ddb8\n\t", "DUALANTENNAHEADINGA,USB3,0,47.5,FINESTEERING,2107,281624.500,02008000,d426,15824;SOL_COMPUTED,NARROW_FLOAT,-1.000000000,78.385162354,-52.385925293,0.0,193.963928223,180.000000000,\"631T\",19,8,8,8,04,00,20,23*14d467ea\n\t", "DUALANTENNAHEADINGA,USB3,0,47.5,FINESTEERING,2107,281625.000,02008000,d426,15824;SOL_COMPUTED,NARROW_FLOAT,-1.000000000,78.697448730,-55.840881348,0.0,201.517425537,180.000000000,\"631T\",20,8,8,8,04,00,20,23*2125c3e9\n\t", "DUALANTENNAHEADINGA,USB3,0,50.0,FINESTEERING,2107,281625.500,02008000,d426,15824;SOL_COMPUTED,NARROW_FLOAT,-1.000000000,76.255996704,-44.440551758,0.0,192.652679443,180.000000000,\"631T\",21,8,8,8,04,00,20,23*2ef6fdf0\n\t", "DUALANTENNAHEADINGA,USB3,0,50.0,FINESTEERING,2107,281626.000,02008000,d426,15824;SOL_COMPUTED,NARROW_FLOAT,-1.000000000,76.051048279,-42.751831055,0.0,190.193801880,180.000000000,\"631T\",19,8,8,8,04,00,20,23*71df93c1\n\t", "DUALANTENNAHEADINGA,USB3,0,49.0,FINESTEERING,2107,281627.000,02000000,d426,15824;SOL_COMPUTED,NARROW_FLOAT,-1.000000000,74.827011108,-47.434204102,0.0,215.584564209,180.000000000,\"631T\",20,6,6,6,04,00,20,03*11cc19a9\n\t", "DUALANTENNAHEADINGA,USB3,0,50.0,FINESTEERING,2107,281627.500,02000000,d426,15824;SOL_COMPUTED,NARROW_FLOAT,-1.000000000,76.736885071,-60.461914063,0.0,257.944244385,180.000000000,\"631T\",20,6,6,6,04,00,20,03*64121f5a\n\t", "DUALANTENNAHEADINGA,USB3,0,50.0,FINESTEERING,2107,281628.000,02000000,d426,15824;SOL_COMPUTED,NARROW_FLOAT,-1.000000000,76.336128235,-57.847045898,0.0,256.018859863,180.000000000,\"631T\",20,6,6,6,04,00,20,03*cae9a6c4\n\t", "DUALANTENNAHEADINGA,USB3,0,49.0,FINESTEERING,2107,281628.500,02000000,d426,15824;SOL_COMPUTED,NARROW_FLOAT,-1.000000000,75.922164917,-51.811248779,0.0,196.475540161,180.000000000,\"631T\",21,6,6,6,04,00,20,03*71a30e30\n\t", "DUALANTENNAHEADINGA,USB3,0,49.0,FINESTEERING,2107,281629.000,02000000,d426,15824;SOL_COMPUTED,NARROW_FLOAT,-1.000000000,75.688812256,-51.816131592,0.0,200.071166992,180.000000000,\"631T\",21,6,6,6,04,00,20,03*05442491\n\t", "DUALANTENNAHEADINGA,USB3,0,47.0,FINESTEERING,2107,281629.500,02000000,d426,15824;SOL_COMPUTED,NARROW_FLOAT,-1.000000000,76.706954956,-45.822814941,0.0,158.336380005,180.000000000,\"631T\",21,7,7,6,04,00,20,03*a7b53285\n\t", "DUALANTENNAHEADINGA,USB3,0,47.0,FINESTEERING,2107,281630.000,02000000,d426,15824;SOL_COMPUTED,NARROW_FLOAT,-1.000000000,76.392150879,-45.545715332,0.0,160.233947754,180.000000000,\"631T\",20,7,7,6,04,00,20,03*a337a603\n\t", "DUALANTENNAHEADINGA,USB3,0,50.0,FINESTEERING,2107,281630.500,02000000,d426,15824;SOL_COMPUTED,NARROW_FLOAT,-1.000000000,73.576385498,-34.237976074,0.0,224.892852783,180.000000000,\"631T\",20,7,7,6,04,00,20,03*509d4fa7\n\t", "DUALANTENNAHEADINGA,USB3,0,50.0,FINESTEERING,2107,281631.000,02000000,d426,15824;SOL_COMPUTED,NARROW_FLOAT,-1.000000000,73.801551819,-34.781646729,0.0,227.056274414,180.000000000,\"631T\",20,7,7,6,04,00,20,03*62a89227\n\t", "DUALANTENNAHEADINGA,USB3,0,48.5,FINESTEERING,2107,281631.500,02000000,d426,15824;SOL_COMPUTED,NARROW_FLOAT,-1.000000000,72.331886292,-39.270935059,0.0,208.219329834,180.000000000,\"631T\",20,6,6,6,04,00,20,03*b4f25b02\n\t", "DUALANTENNAHEADINGA,USB3,0,48.5,FINESTEERING,2107,281632.000,02000000,d426,15824;SOL_COMPUTED,NARROW_FLOAT,-1.000000000,72.392997742,-44.277435303,0.0,216.308242798,180.000000000,\"631T\",20,6,6,6,04,00,20,03*f92d3de0\n\t", "DUALANTENNAHEADINGA,USB3,0,50.5,FINESTEERING,2107,281632.500,02000000,d426,15824;SOL_COMPUTED,NARROW_FLOAT,-1.000000000,70.524742126,-43.222106934,0.0,187.663330078,180.000000000,\"631T\",20,6,6,6,04,00,20,03*23e53db0\n\t", "DUALANTENNAHEADINGA,USB3,0,49.5,FINESTEERING,2107,281634.500,02000000,d426,15824;SOL_COMPUTED,NARROW_FLOAT,-1.000000000,74.599754333,-34.968170166,0.0,186.703521729,180.000000000,\"631T\",21,8,8,8,04,00,20,33*c6f47f17\n\t", "DUALANTENNAHEADINGA,USB3,0,49.5,FINESTEERING,2107,281635.000,02000000,d426,15824;SOL_COMPUTED,NARROW_FLOAT,-1.000000000,74.584259033,-34.924865723,0.0,186.240829468,180.000000000,\"631T\",21,8,8,8,04,00,20,33*9c697b75\n\t", "DUALANTENNAHEADINGA,USB3,0,46.5,FINESTEERING,2107,281635.500,02000000,d426,15824;SOL_COMPUTED,NARROW_FLOAT,-1.000000000,67.143241882,-41.090057373,0.0,270.678344727,180.000000000,\"631T\",21,8,8,8,04,00,20,23*92e43030\n\t", "INSPVAXA,USB3,0,46.5,FINESTEERING,2107,281636.050,02000000,471d,15824;INS_ALIGNMENT_COMPLETE,INS_RTKFIXED,37.37125277821,126.72238773089,7.9249,22.3000,-0.0472,0.2751,0.0261,0.033461112,-0.337994912,90.276833598,0.4107,0.2743,0.5040,0.1102,0.0902,0.0747,0.1666,0.1669,5.1095,0f000001,0*fb0d7dd5\n\t", "INSPVAXA,USB3,0,49.0,FINESTEERING,2107,281636.550,02000000,471d,15824;INS_ALIGNMENT_COMPLETE,INS_RTKFIXED,37.37125270683,126.72238933988,7.9258,22.3000,-0.0404,0.2826,0.0202,-0.092396581,-0.312496368,90.344441421,0.4107,0.2743,0.5040,0.1102,0.0902,0.0747,0.1666,0.1669,5.1095,0f000001,0*2ea03c91\n\t", "DUALANTENNAHEADINGA,USB3,0,45.5,FINESTEERING,2107,281638.000,02000000,d426,15824;SOL_COMPUTED,L1_FLOAT,-1.000000000,68.590065002,-38.051055908,0.0,183.932281494,180.000000000,\"631T\",19,6,6,6,04,00,20,03*7caf4eb9\n\t", "DUALANTENNAHEADINGA,USB3,0,46.5,FINESTEERING,2107,281638.500,02000000,d426,15824;SOL_COMPUTED,NARROW_FLOAT,-1.000000000,65.883399963,-37.877685547,0.0,260.404785156,180.000000000,\"631T\",19,6,6,6,04,00,20,03*2dc9451b\n\t", "DUALANTENNAHEADINGA,USB3,0,46.5,FINESTEERING,2107,281639.000,02000000,d426,15824;SOL_COMPUTED,NARROW_FLOAT,-1.000000000,66.000267029,-38.685607910,0.0,260.610321045,180.000000000,\"631T\",20,6,6,6,04,00,20,03*4d0efe6f\n\t", "DUALANTENNAHEADINGA,USB3,0,48.5,FINESTEERING,2107,281639.500,02000000,d426,15824;SOL_COMPUTED,L1_FLOAT,-1.000000000,75.249496460,-42.510375977,0.0,208.045684814,180.000000000,\"631T\",21,6,6,6,04,00,20,03*5f68b654\n\t", "INSPVAXA,USB3,0,48.5,FINESTEERING,2107,281640.050,02000000,471d,15824;INS_ALIGNMENT_COMPLETE,INS_RTKFIXED,37.37125214763,126.72240056337,7.9297,22.3000,-0.0135,0.2579,0.0068,-0.286062471,-0.323666659,89.847152280,0.4125,0.2764,0.5060,0.1103,0.0900,0.0751,0.1666,0.1668,5.0988,0f000001,0*ba23ac07\n\t", "INSPVAXA,USB3,0,48.0,FINESTEERING,2107,281640.550,02000000,471d,15824;INS_ALIGNMENT_COMPLETE,INS_RTKFIXED,37.37125209177,126.72240219164,7.9302,22.3000,-0.0088,0.2910,0.0070,-0.402825577,-0.342049421,89.793656004,0.4125,0.2764,0.5060,0.1103,0.0900,0.0751,0.1666,0.1668,5.0988,0f000001,0*83e377ec\n\t", "INSPVAXA,USB3,0,49.5,FINESTEERING,2107,281643.050,02000000,471d,15824;INS_ALIGNMENT_COMPLETE,INS_RTKFIXED,37.37125177239,126.72241029930,7.9253,22.3000,-0.0184,0.2626,0.0057,-0.672263501,-0.094085877,89.482974840,0.4115,0.2769,0.5079,0.1098,0.0898,0.0750,0.1665,0.1668,5.0987,0f000001,0*08f45476\n\t", "INSPVAXA,USB3,0,45.0,FINESTEERING,2107,281644.050,02000000,471d,15824;INS_ALIGNMENT_COMPLETE,INS_RTKFIXED,37.37125163862,126.72241353138,7.9238,22.3000,-0.0195,0.2934,0.0047,-0.764058138,0.046945351,89.556014373,0.4117,0.2771,0.5083,0.1098,0.0898,0.0750,0.1665,0.1667,5.0999,0f000001,0*ca60484a\n\t", "INSPVAXA,USB3,0,49.0,FINESTEERING,2107,281644.550,02000000,471d,15824;INS_ALIGNMENT_COMPLETE,INS_RTKFIXED,37.37125159291,126.72241516710,7.9252,22.3000,-0.0125,0.2656,0.0050,-0.825704601,0.105733929,89.608837523,0.4117,0.2771,0.5083,0.1098,0.0898,0.0750,0.1665,0.1667,5.0999,0f000001,0*afd891ca\n\t", "INSPVAXA,USB3,0,49.0,FINESTEERING,2107,281645.050,02000000,471d,15824;INS_ALIGNMENT_COMPLETE,INS_RTKFIXED,37.37125153841,126.72241684941,7.9264,22.3000,-0.0138,0.2766,0.0005,-0.782015483,0.115845462,89.701566718,0.4112,0.2772,0.5084,0.1097,0.0898,0.0750,0.1665,0.1667,5.1015,0f000001,0*e301f266\n\t", "INSPVAXA,USB3,0,51.0,FINESTEERING,2107,281646.050,02000000,471d,15824;INS_ALIGNMENT_COMPLETE,INS_RTKFIXED,37.37125141044,126.72242010916,7.9241,22.3000,-0.0145,0.2894,0.0046,-0.683948152,-0.106427214,89.829684662,0.4110,0.2773,0.5083,0.1096,0.0899,0.0750,0.1665,0.1667,5.1032,0f000001,0*7e3f8e98\n\t", "INSPVAXA,USB3,0,50.5,FINESTEERING,2107,281648.550,02000000,471d,15824;INS_ALIGNMENT_COMPLETE,INS_RTKFIXED,37.37125104211,126.72242819820,7.9192,22.3000,-0.0057,0.2779,0.0043,-0.865746254,0.658403910,90.332036751,0.4101,0.2775,0.5080,0.1095,0.0899,0.0749,0.1664,0.1667,5.1060,0f000001,0*c1bd000c\n\t", "INSPVAXA,USB3,0,47.0,FINESTEERING,2107,281649.050,02000000,471d,15824;INS_ALIGNMENT_COMPLETE,INS_RTKFIXED,37.37125095950,126.72242975720,7.9195,22.3000,-0.0170,0.2957,0.0033,-0.943502690,0.808287959,90.436788993,0.4102,0.2776,0.5078,0.1095,0.0899,0.0749,0.1664,0.1667,5.1072,0f000001,0*5974bd17\n\t", "INSPVAXA,USB3,0,47.0,FINESTEERING,2107,281649.550,02000000,471d,15824;INS_ALIGNMENT_COMPLETE,INS_RTKFIXED,37.37125085766,126.72243133912,7.9203,22.3000,-0.0165,0.2929,0.0110,-0.815482674,0.895195605,90.550000781,0.4102,0.2776,0.5078,0.1095,0.0899,0.0749,0.1664,0.1667,5.1072,0f000001,0*975e6869\n\t", "INSPVAXA,USB3,0,47.0,FINESTEERING,2107,281650.050,02000000,471d,15824;INS_ALIGNMENT_COMPLETE,INS_RTKFIXED,37.37125074410,126.72243299345,7.9208,22.3000,-0.0194,0.2944,0.0151,-0.654661826,0.805584356,90.730688305,0.4111,0.2776,0.5078,0.1096,0.0901,0.0749,0.1664,0.1667,5.1084,0f000001,0*7ee54a6b\n\t", "INSPVAXA,USB3,0,49.5,FINESTEERING,2107,281650.550,02000000,471d,15824;INS_ALIGNMENT_COMPLETE,INS_RTKFIXED,37.37125062801,126.72243464345,7.9218,22.3000,-0.0206,0.2968,0.0101,-0.581641852,0.404768185,90.963959440,0.4111,0.2776,0.5078,0.1096,0.0901,0.0749,0.1664,0.1667,5.1084,0f000001,0*f2a4c14e\n\t", "INSPVAXA,USB3,0,49.5,FINESTEERING,2107,281651.050,02000000,471d,15824;INS_ALIGNMENT_COMPLETE,INS_RTKFIXED,37.37125051285,126.72243625014,7.9235,22.3000,-0.0268,0.3045,0.0175,-0.662592503,0.202583400,91.123013334,0.4115,0.2778,0.5076,0.1098,0.0901,0.0749,0.1663,0.1667,5.1090,0f000001,0*216f234f\n\t", "INSPVAXA,USB3,0,45.5,FINESTEERING,2107,281652.050,02000000,471d,15824;INS_ALIGNMENT_COMPLETE,INS_RTKFIXED,37.37125028624,126.72243951930,7.9245,22.3000,-0.0369,0.2898,0.0166,-0.721183306,0.056680654,91.387520198,0.4416,0.2813,0.5208,0.1150,0.0908,0.0760,0.1664,0.1673,5.1091,0f000001,0*25228c2c\n\t", "INSPVAXA,USB3,0,47.5,FINESTEERING,2107,281653.050,02000000,471d,15824;INS_ALIGNMENT_COMPLETE,INS_RTKFIXED,37.37125003154,126.72244272682,7.9262,22.3000,-0.0470,0.2934,0.0145,-0.464349418,0.202545011,91.639204054,0.4699,0.2842,0.5361,0.1187,0.0913,0.0769,0.1664,0.1677,5.1090,0f000001,0*2b109b71\n\t", "INSPVAXA,USB3,0,47.5,FINESTEERING,2107,281653.550,02000000,471d,15824;INS_ALIGNMENT_COMPLETE,
